vi "m1m3_logEvent_GyroWarning.vi"(8 "error in (no error)":errorcluster, 11 "logevent_GyroWarning_Ctl":T1) -> (0 "error out":errorcluster, 2 "function return":i32, 3 "logevent_GyroWarning_Ctl out":T1)   [LabVIEW 2016, in "SALLV_m1m3.lvlib"]
doc: "int m1m3_shm_logEvent_GyroWarningLV(m1m3_logevent_GyroWarningLV *logevent_GyroWarning_Ctl );"
uses:
  SALLV_m1m3.lvlib
  DataTypes/logevent_GyroWarning.ctl
  SALLV_m1m3.so
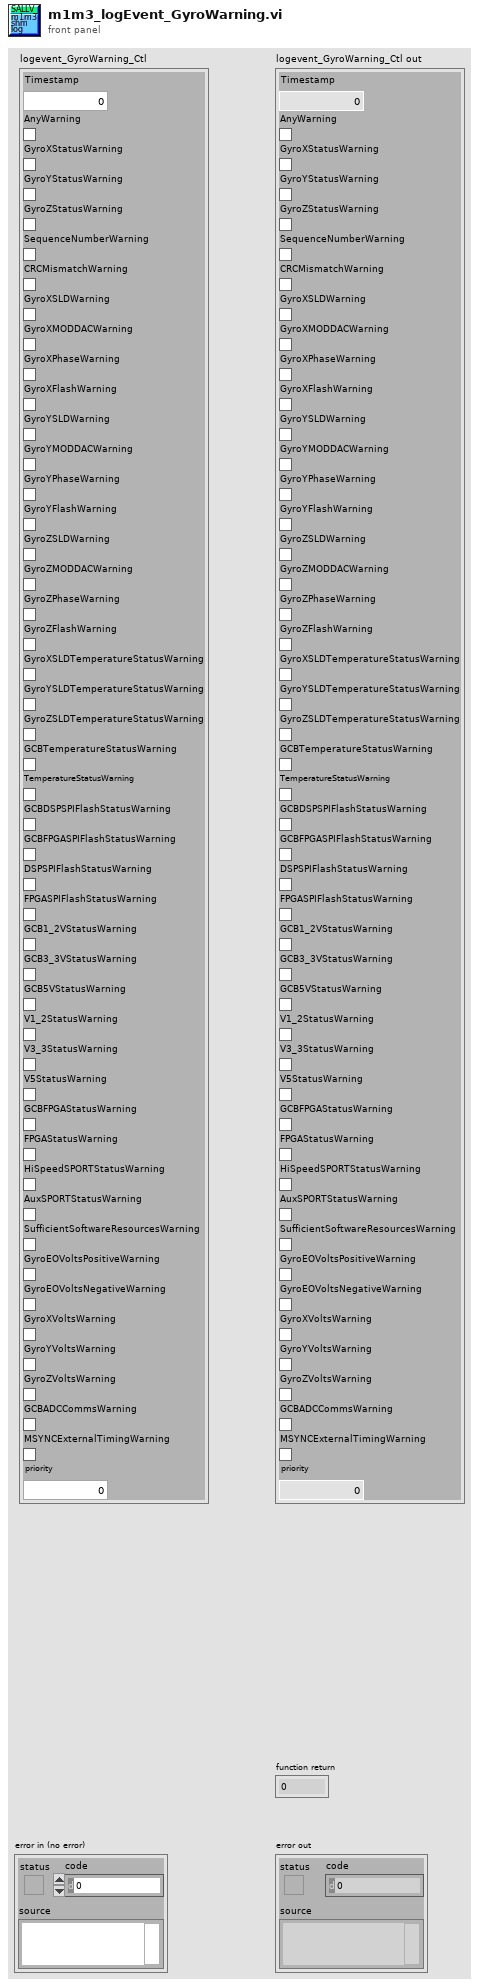
[diagram p1: front panel]
types:
  T1 = typedef "SALLV_m1m3.lvlib/logevent_GyroWarning.ctl" = cluster{"Timestamp":dbl, "AnyWarning":bool, "GyroXStatusWarning":bool, "GyroYStatusWarning":bool, "GyroZStatusWarning":bool, "SequenceNumberWarning":bool, "CRCMismatchWarning":bool, "GyroXSLDWarning":bool, "GyroXMODDACWarning":bool, "GyroXPhaseWarning":bool, "GyroXFlashWarning":bool, "GyroYSLDWarning":bool, "GyroYMODDACWarning":bool, "GyroYPhaseWarning":bool, "GyroYFlashWarning":bool, "GyroZSLDWarning":bool, "GyroZMODDACWarning":bool, "GyroZPhaseWarning":bool, "GyroZFlashWarning":bool, "GyroXSLDTemperatureStatusWarning":bool, "GyroYSLDTemperatureStatusWarning":bool, "GyroZSLDTemperatureStatusWarning":bool, "GCBTemperatureStatusWarning":bool, "TemperatureStatusWarning":bool, "GCBDSPSPIFlashStatusWarning":bool, "GCBFPGASPIFlashStatusWarning":bool, "DSPSPIFlashStatusWarning":bool, "FPGASPIFlashStatusWarning":bool, "GCB1_2VStatusWarning":bool, "GCB3_3VStatusWarning":bool, "GCB5VStatusWarning":bool, "V1_2StatusWarning":bool, "V3_3StatusWarning":bool, "V5StatusWarning":bool, "GCBFPGAStatusWarning":bool, "FPGAStatusWarning":bool, "HiSpeedSPORTStatusWarning":bool, "AuxSPORTStatusWarning":bool, "SufficientSoftwareResourcesWarning":bool, "GyroEOVoltsPositiveWarning":bool, "GyroEOVoltsNegativeWarning":bool, "GyroXVoltsWarning":bool, "GyroYVoltsWarning":bool, "GyroZVoltsWarning":bool, "GCBADCCommsWarning":bool, "MSYNCExternalTimingWarning":bool, "priority":i32}
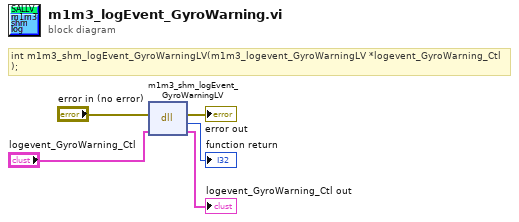
[diagram p0: block diagram]
diagram:
  # "int m1m3_shm_logEvent_GyroWarningLV(m1m3_logevent_GyroWarningLV *logevent_GyroWarning_Ctl );"
  n1 = dll-call lib="opt/CODE/SALLV_m1m3/SALLV_m1m3.*" fn="m1m3_shm_logEvent_GyroWarningLV"(error in="error in (no error)", "logevent_GyroWarning_Ctl"="logevent_GyroWarning_Ctl") -> (error out=→"error out":errorcluster, →"function return":i32, "logevent_GyroWarning_Ctl"=→"logevent_GyroWarning_Ctl out":T1)  [unwired: 2 in, 1 out]
